vi "3D Model Init (SubVI).vi"(11 "STL File Path":path=path "C:/Users/Marcin_2/Documents/Quadrocopter/QuadroTwins-master/QuadroController LabView/quadro.stl") -> (0 "error out":errorcluster, 3 "SceneObject out":refnum<vi>)   [LabVIEW 2012]
uses:
  <vilib>/picture/3D Picture Control/NI_3D Picture Control.lvlib
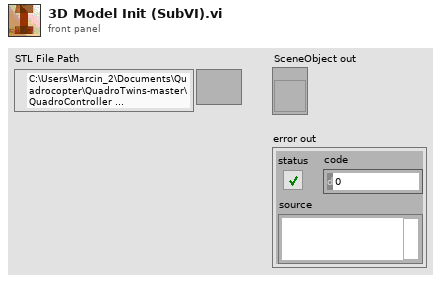
[diagram p1: front panel]
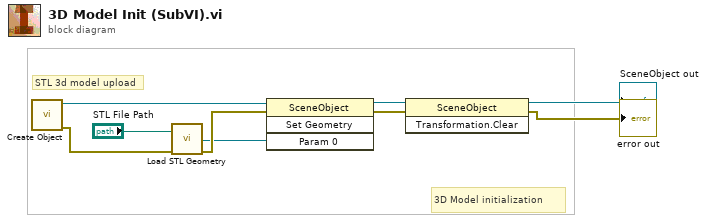
[diagram p0: block diagram]
diagram:
  # "3D Model initialization"
  # "STL 3d model upload"
  n1 = call <vilib>:"Create Object.vi"() -> ("error out"=w2:errorcluster, "Scene:New Object"=w4:refnum<vi>)  [unwired: 2 in, 8 out]
  n2 = call <vilib>:"Load STL Geometry.vi"("error in (no error)"=w2, "Model File"="STL File Path") -> ("error out"=w5:errorcluster, "New Mesh Refnum"=w3:refnum<vi>)  [unwired: 8 out]
  n3 = invoke class="SceneObject" method="Set Geometry"(reference=w4, error in=w5, "Param 0"=w3) -> (reference out=w6:refnum<vi>, error out=w7:errorcluster)  [unwired: 1 in, 2 out]
  n4 = invoke class="SceneObject" method="Transformation.Clear"(reference=w6, error in=w7) -> (reference out=→"SceneObject out":refnum<vi>, error out=→"error out":errorcluster)  [unwired: 1 in, 1 out]
